vi "ReadClassAttribute.vi"(5 "error in (no error)":errorcluster) -> (19 "error out":errorcluster)   [LabVIEW 2020, in "G#MethodTemplates.lvclass"]
uses:
  <vilib>/addons/_AddQ/G#Templates/G#MethodTemplates/G#MethodTemplates.lvclass
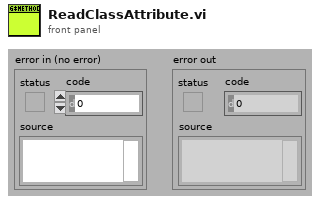
[diagram p1: front panel]
types:
  T1 = typedef "G#MethodTemplates.lvclass/ClassAttributes.ctl" = cluster{"Dummy":bool}
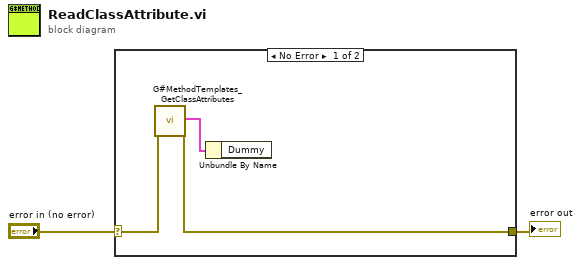
[diagram p0: block diagram]
diagram:
  n1 = case shown="No Error" "error in (no error)" {
    selector: "error in (no error)" -> [w5 w6]
    tunnel: [w4 w6] -> w1
    frame No Error {
      n2 = call <vilib>:"G#MethodTemplates_GetClassAttributes.vi"("error in (no error)"=w5) -> ("class attributes"=w3:T1, "error out"=w4:errorcluster)  [unwired: 15 in, 2 out]
      n3 = Unbundle By Name(w3) -> ()  [unwired: 1 out]
    }
    frame Error {
    }
  }
  "error out" <- w1
